vi "[WLC] Calculate Contour Length.vi"(1 "Temperature (K)":dbl=298.0, 2 "Persistence Length (nm)":dbl, 3 "Extension (nm)":dbl, 4 "Force (pN)":dbl) -> (0 "Contour Length (nm)":dbl)   [LabVIEW 2013]
uses:
  <vilib>/Analysis/polynomials.llb/Polynomial Roots (DBL).vi
  <vilib>/Analysis/NI_AALPro.lvlib
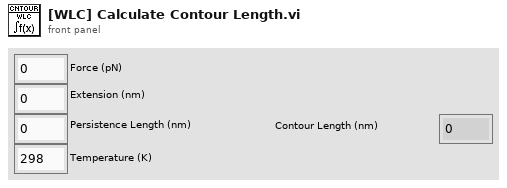
[diagram p1: front panel]
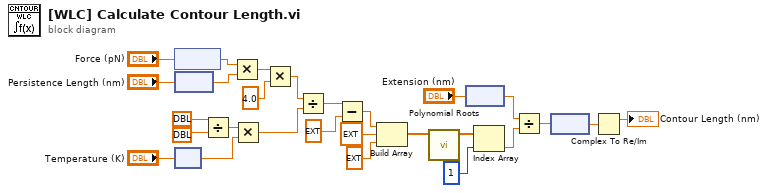
[diagram p0: block diagram]
diagram:
  n1 = node("Force (pN)") -> (w10:dbl[unit])
  n2 = node("Persistence Length (nm)") -> (w9:dbl[unit])
  n3 = node("Temperature (K)") -> (w23:dbl[unit])
  n4 = Divide(x=ext[unit] 8.314472, y=ext[unit] 6.0221415e+23) -> (x/y=w25:ext[unit])
  n5 = Multiply(x=w10, y=w9) -> (x*y=w22:dbl[unit])
  n6 = Multiply(x=w25, y=w23) -> (x*y=w13:ext[unit])
  n7 = Multiply(x=w22, y=4.0) -> (x*y=w20:dbl[unit])
  n8 = Divide(x=w20, y=w13) -> (x/y=w19:ext)
  n9 = Subtract(x=w19, y=ext 3.0) -> (x-y=w17:ext)
  n10 = Build Array(w17, ext -2.0 ("y"), ext 1.0 ("y")) -> (w14:ext[])
  n11 = call-poly <vilib>:"Polynomial Roots.vi"("P(x)"=w14) -> ("Roots"=w7:cdb[])  [unwired: 9 in, 1 out]
  n12 = node("Extension (nm)") -> (w5:dbl[unit])
  n13 = Index Array(array=w7, index=1) -> (element=w4:cdb)
  n14 = Divide(x=w5, y=w4) -> (x/y=w3:cdb[unit])
  n15 = node(w3) -> (w2:cdb)
  n16 = Complex To Re/Im(x + iy=w2) -> (x=→"Contour Length (nm)":dbl)  [unwired: 1 out]
